vi "EnumerateElements.vi"(8 "error in (no error)":errorcluster, 10 "Qualified Name":string, 11 "ConfigManagerCollection in":refnum<class "ConfigManagerCollection.lvclass">) -> (0 "error out":errorcluster, 2 "keys":string[](array[string]), 3 "ConfigManagerCollection out":refnum<class "ConfigManagerCollection.lvclass">)   [LabVIEW 2013, in "SMOConfig.lvlib" / "ConfigManagerCollection.lvclass"]
uses:
  ConfigManagerCollection.lvclass
  Manager/ConfigManager.lvclass
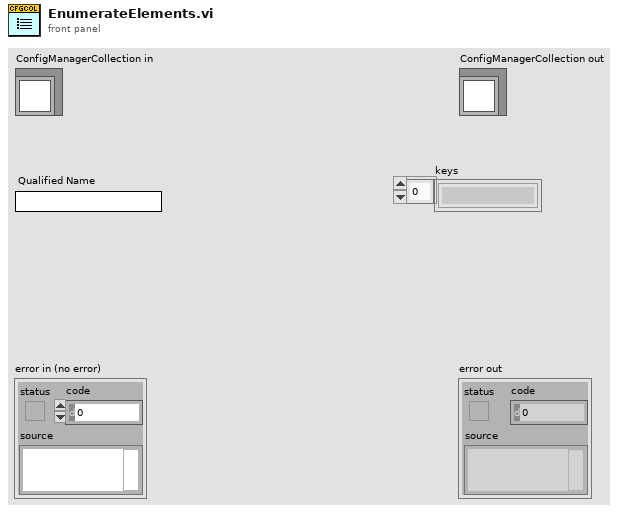
[diagram p1: front panel]
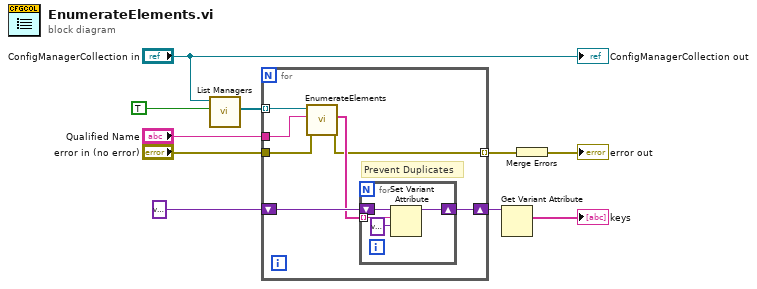
[diagram p0: block diagram]
diagram:
  n1 = call-dynamic "List Managers.vi"("Include Cache? (F)"=TRUE, "SMOConfigManagerCollection in"="ConfigManagerCollection in") -> ("List"=w9:refnum<class "ConfigManager.lvclass">[])  [unwired: 8 in, 1 out]
  n2 = for {
    tunnel: w9 -> [w17] mode=indexing
    tunnel: "Qualified Name" -> [w16]
    tunnel: "error in (no error)" -> [w15]
    shift-right: [w13] -> w5
    shift-left: variant ("variant") -> [w14]
    tunnel: [w11] -> w3 mode=indexing
    # "Prevent Duplicates"
    n3 = call-dynamic "EnumerateElements.vi"("error in (no error)"=w15, "Qualified Name"=w16, "ConfigManager in"=w17) -> ("error out"=w11:errorcluster, "keys"=w12:string[])  [unwired: 6 in, 1 out]
    n4 = for {
      tunnel: w12 -> [w20] mode=indexing
      shift-right: [w18] -> w13
      shift-left: w14 -> [w21]
      n5 = Set Variant Attribute(Variant=w21, name=w20, value=variant ("variant")) -> (Variant out=w18:variant)  [unwired: 1 in, 2 out]
    }
  }
  n6 = Get Variant Attribute(Variant=w5) -> (names=→"keys":string[])  [unwired: 3 in, 3 out]
  n7 = Merge Errors(w3) -> (→"error out":errorcluster)
  "ConfigManagerCollection out" <- "ConfigManagerCollection in"
